vi "Balance.vi"() -> (19 "Done":bool)   [LabVIEW 2020]
uses:
  <vilib>/Rock Robotics/WPI/Utilities/WPI_GetSetVariantRefNum.vi
  Robot Global Data.vi
  <vilib>/Rock Robotics/WPI/RobotDrive/WPI_RobotDriveArcadeDrive_Standard(NoSaturation).vi
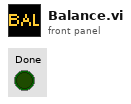
[diagram p1: front panel]
types:
  T1 = typedef "WPI_RobotDriveDevRef.ctl" = cluster{"DevStatus":errorcluster, "Motors[]":T2[], "Square Inputs":bool, "Max Output":dbl}
  T2 = typedef "WPI_MotorControlDeviceRef.ctl" = cluster{"DeviceStatus":errorcluster, "Type":T3, "PWM":cluster{"PWM Channel":T4, "DeadBand":T5}, "CAN":cluster{"Device Number":u8, "SetOutput VI Ref":variant, "GetOutput VI Ref":variant, "Enable VI Ref":variant, "Disable VI Ref":variant, "Data":variant}, "Invert":bool, "DIO PWM":cluster{"PWM \"Enable\" Channel":T4, "DIOChannel":T6, "PWM Rate":dbl}}
  T3 = typedef "WPI_MotorControlType.ctl" = enum16{"PWM", "CAN", "DIO PWM"}
  T4 = typedef "FPGA_DIOPWMChannel.ctl" = enum8{"PWM 0", "PWM 1", "PWM 2", "PWM 3", "PWM 4", "PWM 5", "PWM 6", "PWM 7", "PWM 8", "PWM 9", "PWM MXP 0", "PWM MXP 1", "PWM MXP 2", "PWM MXP 3", "PWM MXP 4", "PWM MXP 5", "PWM MXP 6", "PWM MXP 7", "PWM MXP 8", "PWM MXP 9", "Invalid"}
  T5 = typedef "WPI_PWMDeadband.ctl" = cluster{"Name":string, "maxPositivePwm":i32, "minPositivePwm":i32, "centerPwm":i32, "maxNegativePwm":i32, "minNegativePwm":i32, "angularRange":u16}
  T6 = typedef "FPGA_DIOChannel.ctl" = enum8{"DIO 0", "DIO 1", "DIO 2", "DIO 3", "DIO 4", "DIO 5", "DIO 6", "DIO 7", "DIO 8", "DIO 9", "DIO MXP 0", "DIO MXP 1", "DIO MXP 2", "DIO MXP 3", "DIO MXP 4", "DIO MXP 5", "DIO MXP 6", "DIO MXP 7", "DIO MXP 8", "DIO MXP 9", "DIO MXP 10", "DIO MXP 11", "DIO MXP 12", "DIO MXP 13", "DIO MXP 14", "DIO MXP 15", "SPI Port CS1", "SPI Port CS2", "SPI Port CS3", "SPI Port MISO", "SPI Port MOSI", "Invalid"}
  T7 = typedef "ADIS16470 Device Reference.ctl" = cluster{"DevStatus":errorcluster, "Hardware Config":T8, "Calibration Complete":refnum<notifier>, "Status Reference":refnum<data-value>, "Data Reference":refnum<data-value>, "Sychronous Process VI":T11, "Cmd FIFO":refnum<k33>, "Source":T12, "Data FIFO":refnum<k33>, "Calibration Time (ms)":u32, "Data Reference":refnum<data-value>}
  T8 = typedef "ADIS16470 Hardware Configuration.ctl" = cluster{"SPI Clock Rate (Hz)":dbl, "IMU SPI Mode (3)":T9, "IMU Reset Pin":T6, "IMU SPI Bus":T10, "IMU Data Ready Pin":T6, "Stall Config":cluster{"Pow2BytesPerRead":u8, "StallTicks":u16, "CsToSclkTicks":u8}}
  T9 = typedef "WPI_SPIMode.ctl" = enum16{"Mode 0 (Clk Idle Low,Sample on Leading)", "Mode 1 (Clk Idle Low,Sample on Trailing)", "Mode 2 (Clk Idle High,Sample on Leading)", "Mode 3 (Clk Idle High,Sample on Trailing)"}
  T10 = typedef "spi_bus.ctl" = enum16{"SPI On-Board, CS0", "SPI On-Board, CS1", "SPI On-Board, CS2", "SPI On-Board, CS3", "SPI MXP", "Invalid"}
  T11 = typedef "ADIS16470 Process.ctl" = refnum<vi>
  T12 = typedef "FPGA_CounterEncoderSourceConvertionLVSourceType.ctl" = cluster{"DevStatus":errorcluster, "AnalogTriggerMode?":bool, "DigitalMode":cluster{"DIO Channel":T13}, "AnalogTriggerMode":cluster{"AnalogTriggerIndex":T14, "OutputType":T15}}
  T13 = typedef "FPGA_DIODigitalSourceChannel.ctl" = enum8{"DIO 0", "DIO 1", "DIO 2", "DIO 3", "DIO 4", "DIO 5", "DIO 6", "DIO 7", "DIO 8", "DIO 9", "DIO MXP 0", "DIO MXP 1", "DIO MXP 2", "DIO MXP 3", "DIO MXP 4", "DIO MXP 5", "DIO MXP 6", "DIO MXP 7", "DIO MXP 8", "DIO MXP 9", "DIO MXP 10", "DIO MXP 11", "DIO MXP 12", "DIO MXP 13", "DIO MXP 14", "DIO MXP 15", "SPI Port CS1", "SPI Port CS2", "SPI Port CS3", "SPI Port MISO", "SPI Port MOSI", "Disabled"}
  T14 = typedef "FPGA_AnalogTriggerIndex.ctl" = enum8{"Trig 0", "Trig 1", "Trig 2", "Trig 3", "Trig 4", "Trig 5", "Trig 6", "Trig 7", "Invalid"}
  T15 = typedef "FPGA_AnalogTriggerOutType.ctl" = enum16{"InWindow", "TriggerState", "Rising", "Falling"}
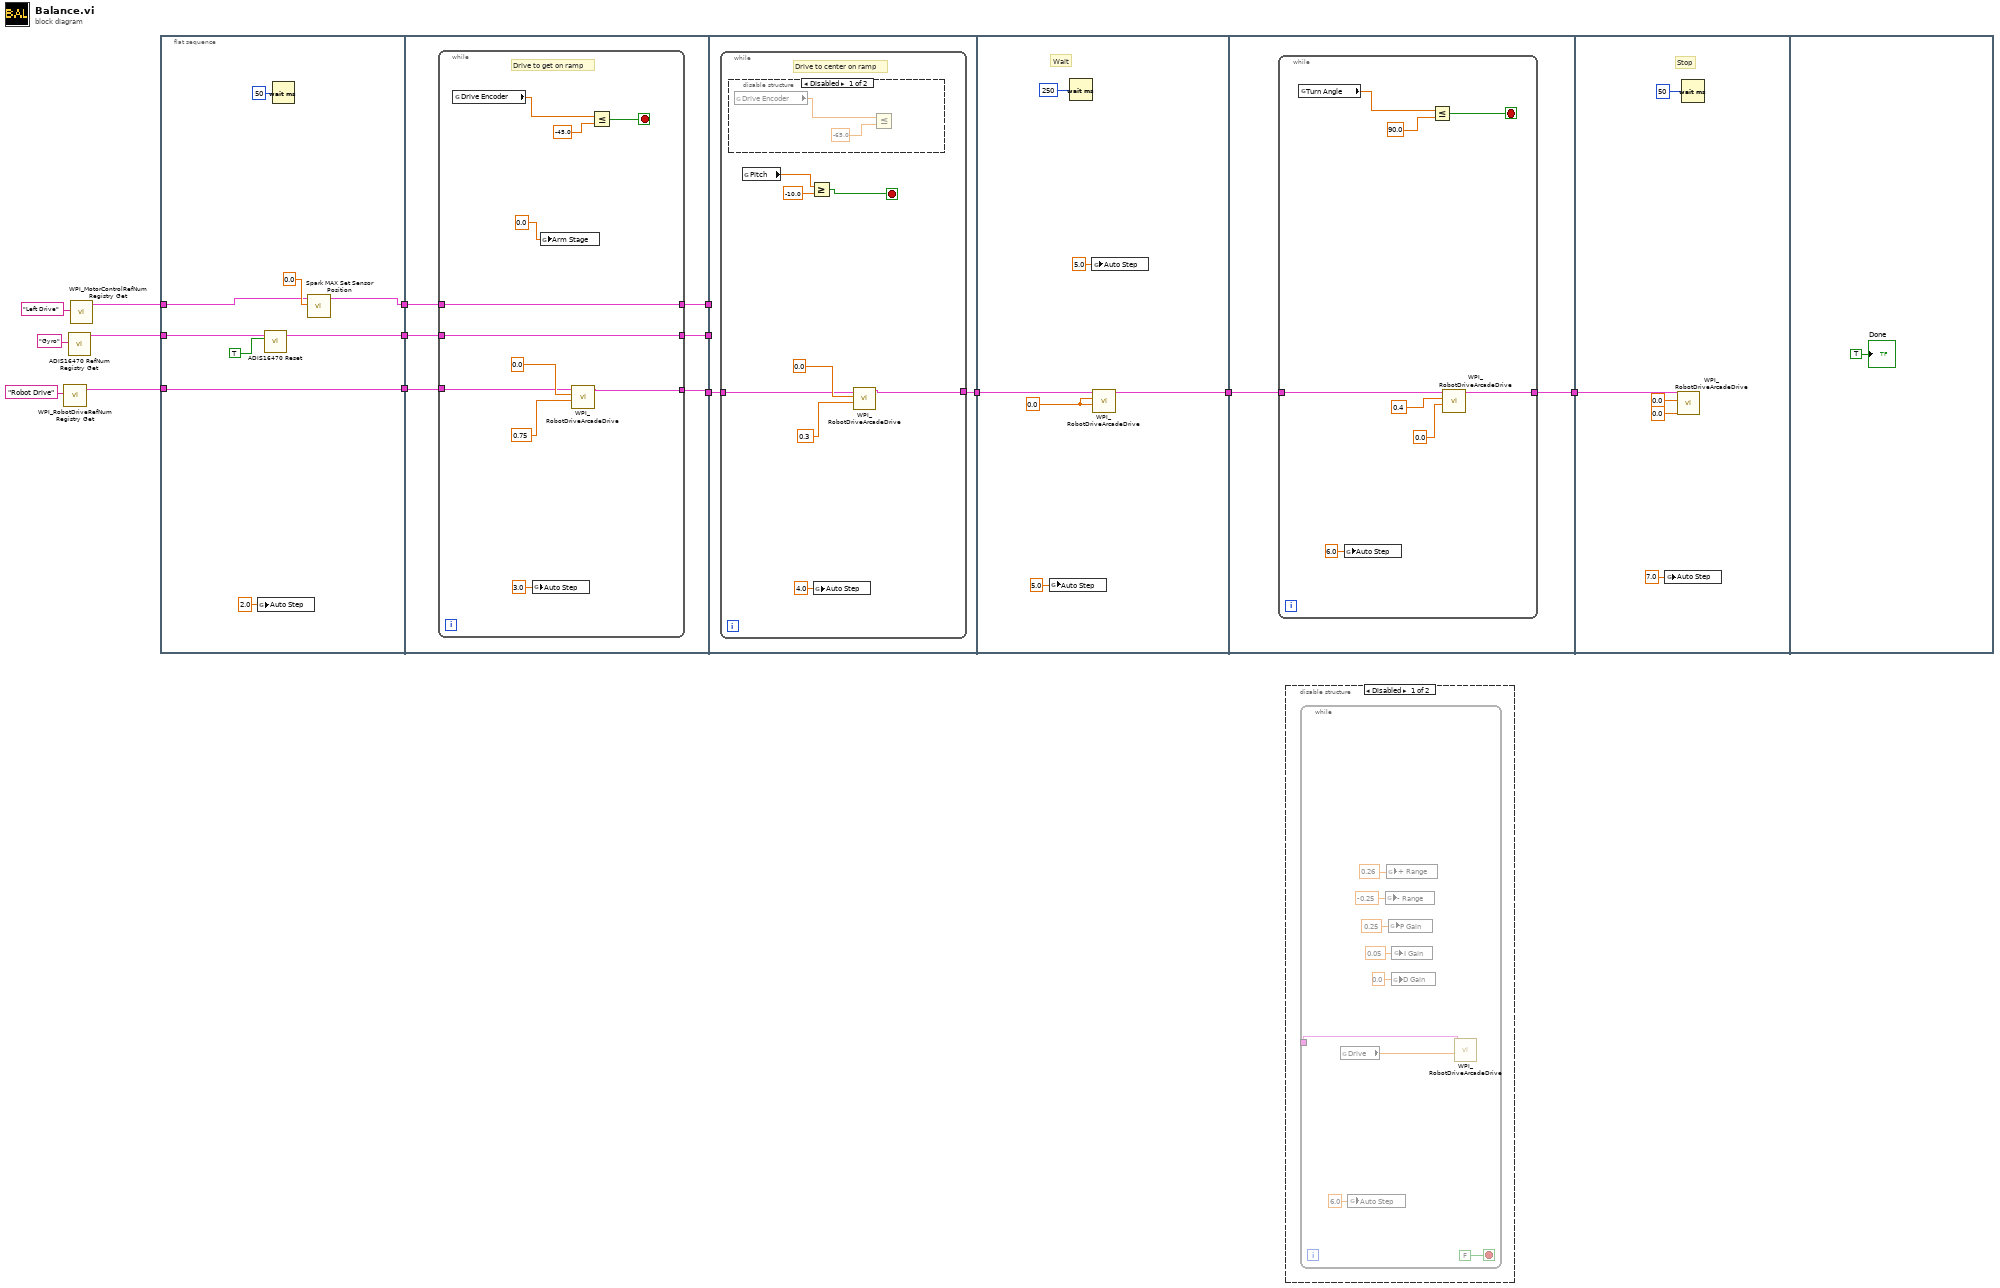
[diagram p0: block diagram]
diagram:
  n1 = call <vilib>:"WPI_RobotDriveRefNum Registry Get.vi"("refnum name"="Robot Drive") -> ("RobotDriveDevRef"=w2:T1)  [unwired: 9 in, 1 out]
  n2 = call <vilib>:"ADIS16470 RefNum Registry Get.vi"("refnum name"="Gyro") -> ("ADIS16470DevRef out"=w3:T7)  [unwired: 9 in, 1 out]
  n3 = call <vilib>:"WPI_MotorControlRefNum Registry Get.vi"("refnum name"="Left Drive") -> ("MotorControlDevRef"=w4:T2)  [unwired: 9 in, 1 out]
  n4 = flat-sequence {
    tunnel: [w24] -> w15
    tunnel: [w21] -> w14
    tunnel: w2 -> [w24]
    tunnel: w3 -> [w20]
    tunnel: w4 -> [w16]
    tunnel: [w17] -> w13
    tunnel: w15 -> [w28]
    tunnel: [w27] -> w12
    tunnel: w14 -> [w29]
    tunnel: [w26] -> w11
    tunnel: [w25] -> w10
    tunnel: w13 -> [w30]
    tunnel: w12 -> [w43]
    tunnel: w11 -> [_]
    tunnel: w10 -> [_]
    tunnel: [w42] -> w9
    tunnel: [w56] -> w8
    tunnel: w9 -> [w57]
    tunnel: w8 -> [w61]
    tunnel: [w60] -> w1
    tunnel: w1 -> [w73]
    frame #0 {
      n5 = global write "Robot Global Data.vi" "Auto Step"(2.0 ("Auto Step")) -> ()
      n6 = call <vilib>:"ADIS16470 Reset.vi"("Reset? (T)"=TRUE, "ADIS16470DevRef"=w20) -> ("ADIS16470DevRef"=w21:T7)  [unwired: 8 in, 1 out]
      n7 = Wait (ms)(milliseconds to wait=u32 50) -> ()  [unwired: 1 out]
      n8 = call <vilib>:"Spark MAX Set Sensor Position.vi"("Position"=0.0, "MotorControlDeviceRef"=w16) -> ("MotorControlDeviceRef"=w17:T2)  [unwired: 8 in, 1 out]
    }
    frame #1 {
      n9 = while {
        tunnel: w28 -> [w39]
        tunnel: [w34] -> w27
        tunnel: [w33] -> w25
        tunnel: w29 -> [w33]
        tunnel: [w32] -> w26
        tunnel: w30 -> [w32]
        stop <- w36 stop-if-true
        # "Drive to get on ramp"
        n10 = global read "Robot Global Data.vi" "Drive Encoder"() -> (w38:dbl)
        n11 = global write "Robot Global Data.vi" "Auto Step"(3.0 ("Auto Step")) -> ()
        n12 = global write "Robot Global Data.vi" "Arm Stage"(0.0 ("Arm Stage")) -> ()
        n13 = call-poly <vilib>:"WPI_RobotDriveArcadeDrive.vi"("Y axis value"=0.75, "X axis value"=0.0, "RobotDriveDevRef"=w39) -> ("RobotDriveDevRef"=w34:T1)  [unwired: 6 in, 2 out]
        n14 = Less Or Equal?(x=w38, y=-45.0) -> (x <= y?=w36:bool)
      }
    }
    frame #2 {
      n15 = while {
        tunnel: [w49] -> w42
        tunnel: w43 -> [w47]
        stop <- w44 stop-if-true
        # "Drive to center on ramp"
        n16 = disable-structure shown="Disabled" {
          frame Disabled {
            n17 = global read "Robot Global Data.vi" "Drive Encoder"() -> (w53:dbl)
            n18 = Less Or Equal?(x=w53, y=-65.0) -> ()  [unwired: 1 out]
          }
          frame Enabled {
          }
        }
        n19 = global read "Robot Global Data.vi" "Pitch"() -> (w46:dbl)
        n20 = Greater Or Equal?(x=w46, y=-10.0) -> (x >= y?=w44:bool)
        n21 = global write "Robot Global Data.vi" "Auto Step"(4.0 ("Auto Step")) -> ()
        n22 = call-poly <vilib>:"WPI_RobotDriveArcadeDrive.vi"("Y axis value"=0.3, "X axis value"=0.0, "RobotDriveDevRef"=w47) -> ("RobotDriveDevRef"=w49:T1)  [unwired: 6 in, 2 out]
      }
    }
    frame #3 {
      w55 = 0.0 ("X axis value")
      # "Wait"
      n23 = global write "Robot Global Data.vi" "Auto Step"(5.0 ("Auto Step")) -> ()
      n24 = Wait (ms)(milliseconds to wait=u32 250) -> ()  [unwired: 1 out]
      n25 = global write "Robot Global Data.vi" "Auto Step"(5.0 ("Auto Step")) -> ()
      n26 = call-poly <vilib>:"WPI_RobotDriveArcadeDrive.vi"("Y axis value"=w55, "X axis value"=w55, "RobotDriveDevRef"=w57) -> ("RobotDriveDevRef"=w56:T1)  [unwired: 6 in, 2 out]
    }
    frame #4 {
      n27 = while {
        tunnel: w61 -> [w65]
        tunnel: [w62] -> w60
        stop <- w66 stop-if-true
        n28 = global read "Robot Global Data.vi" "Turn Angle"() -> (w68:dbl)
        n29 = global write "Robot Global Data.vi" "Auto Step"(6.0 ("Auto Step")) -> ()
        n30 = Less Or Equal?(x=w68, y=90.0) -> (x <= y?=w66:bool)
        n31 = call-poly <vilib>:"WPI_RobotDriveArcadeDrive.vi"("Y axis value"=0.0, "X axis value"=0.4, "RobotDriveDevRef"=w65) -> ("RobotDriveDevRef"=w62:T1)  [unwired: 6 in, 2 out]
      }
    }
    frame #5 {
      # "Stop"
      n32 = global write "Robot Global Data.vi" "Auto Step"(7.0 ("Auto Step")) -> ()
      n33 = call-poly <vilib>:"WPI_RobotDriveArcadeDrive.vi"("Y axis value"=0.0, "X axis value"=0.0, "RobotDriveDevRef"=w73) -> ()  [unwired: 6 in, 3 out]
      n34 = Wait (ms)(milliseconds to wait=u32 50) -> ()  [unwired: 1 out]
    }
    frame #6 {
      "Done" <- TRUE ("Done")
    }
  }
  n35 = disable-structure shown="Disabled" {
    frame Disabled {
      n36 = while {
        tunnel: _ -> [w77]
        stop <- FALSE stop-if-true
        n37 = global read "Robot Global Data.vi" "Drive"() -> (w84:dbl)
        n38 = global write "Robot Global Data.vi" "Auto Step"(6.0 ("Auto Step")) -> ()
        n39 = global write "Robot Global Data.vi" "- Range"(-0.25 ("- Range")) -> ()
        n40 = global write "Robot Global Data.vi" "+ Range"(0.26 ("+ Range")) -> ()
        n41 = global write "Robot Global Data.vi" "P Gain"(0.25 ("P Gain")) -> ()
        n42 = global write "Robot Global Data.vi" "D Gain"(0.0 ("D Gain")) -> ()
        n43 = global write "Robot Global Data.vi" "I Gain"(0.05 ("I Gain")) -> ()
        n44 = call-poly <vilib>:"WPI_RobotDriveArcadeDrive.vi"("Y axis value"=w84, "RobotDriveDevRef"=w77) -> ()  [unwired: 7 in, 3 out]
      }
    }
    frame Enabled {
    }
  }
